vi "ma_SML Data Packing (complex input) (No State).vi"(6 "reset?":bool, 7 "ma_SML Data Packing (complex input) state":T1, 8 "error in (no error)":errorcluster, 9 "%overlap":dbl format="%.2f", 10 "size":i32, 11 "x":cdb[](array[numeric]) format="%.2f") -> (0 "error out":errorcluster, 1 "data ready?":bool, 3 "y":cdb[](array[numeric]) format="%.2f", 5 "ma_SML Data Packing (complex input) state":T1)   [LabVIEW 2020, in "NI_MAPro.lvlib"]
uses:
  NI_MAPro.lvlib
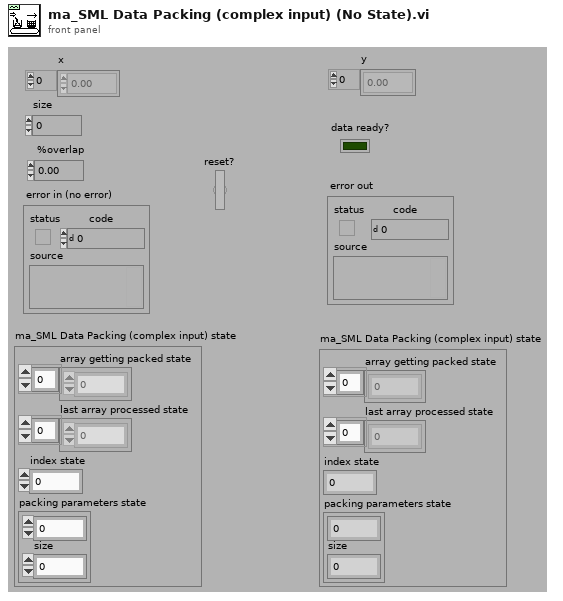
[diagram p1: front panel]
types:
  T1 = cluster{"array getting packed state":cdb[], "last array processed state":cdb[], "index state":i32, "packing parameters state":cluster{i32, "size":i32}}
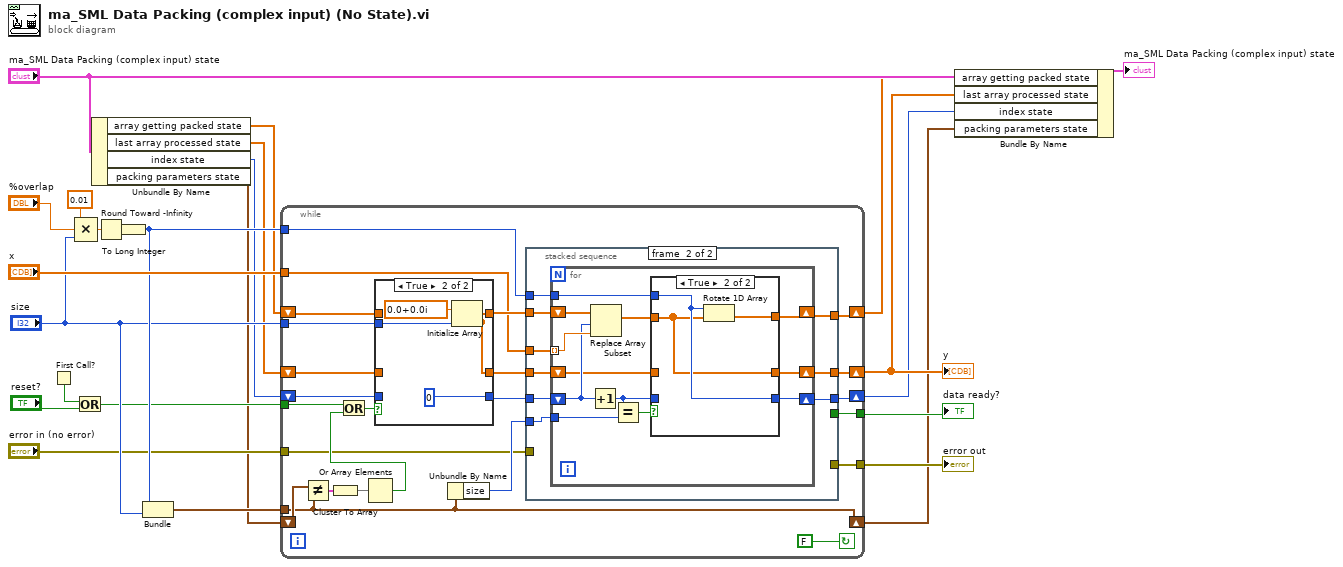
[diagram p0: block diagram]
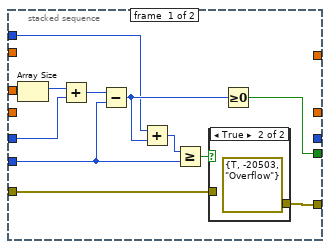
[diagram p2: hidden frame]
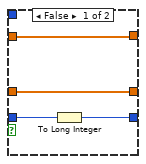
[diagram p4: hidden frame]
diagram:
  n1 = First Call?() -> (First Call?: T/F=w12:bool)
  n2 = Compound Arithmetic op=MULTIPLY(0.01, "%overlap", "size") -> (w24:dbl)
  n3 = Or(x=w12, y="reset?") -> (x .or. y?=w13:bool)
  n4 = Unbundle By Name("ma_SML Data Packing (complex input) state") -> ("array getting packed state"=w8:cdb[], "last array processed state"=w7:cdb[], "index state"=w6:i32, "packing parameters state"=w5:cluster{i32, "size":i32})
  n5 = Round Toward -Infinity(1:w24) -> (0:w21:dbl)
  n6 = To Long Integer(number=w21) -> (32bit integer=w18:i32)
  n7 = Bundle(w18, "size"="size") -> (w20:cluster{i32, "size":i32})  [unwired: 1 out]
  n8 = while {
    tunnel: "error in (no error)" -> [w25]
    tunnel: [w27] -> w14
    tunnel: w13 -> [w32]
    tunnel: [w33] -> w16
    tunnel: w18 -> [w34]
    tunnel: "x" -> [w39]
    tunnel: "size" -> [w43]
    shift-left: w6 -> [w45]
    shift-right: [w35] -> w2
    shift-left: w7 -> [w44]
    shift-right: [w37] -> w3
    shift-left: w8 -> [w42]
    shift-right: [w40] -> w4
    tunnel: w20 -> [w29]
    shift-left: w5 -> [w46]
    shift-right: [w29] -> w1
    stop <- FALSE continue-if-true
    n9 = Not Equal?(x=w46, y=w29) -> (x != y?=w48:cluster{bool, "size":bool})
    n10 = Cluster To Array(cluster=w48) -> (array=w47:bool[])
    n11 = Or Array Elements(Boolean array=w47) -> (logical OR=w31:bool)
    n12 = Or(x=w32, y=w31) -> (x .or. y?=w30:bool)
    n13 = case shown="True" w30 {
      tunnel: [w93 0] -> w36
      tunnel: w45 -> [w93 _]
      tunnel: w44 -> [w92 _]
      tunnel: [w92 w94] -> w38
      tunnel: w43 -> [_ w95]
      tunnel: [w91 w94] -> w41
      tunnel: w42 -> [w91 _]
      frame False {
      }
      frame True {
        n14 = Initialize Array(cdb 0.0+0.0i ("Element Data"), w95) -> (w94:cdb[])
      }
    }
    n15 = Unbundle By Name(w29) -> ("size"=w28:i32)
    n16 = stacked-sequence {
      tunnel: w39 -> [w60 w71]
      tunnel: w41 -> [_ w66]
      tunnel: w36 -> [w59 w67]
      tunnel: w28 -> [w53 w70]
      tunnel: [_ w68] -> w35
      tunnel: [_ w63] -> w37
      tunnel: w38 -> [_ w64]
      tunnel: [_ w65] -> w40
      tunnel: w34 -> [w50 w69]
      tunnel: [w55 _] -> w33
      tunnel: [w56 _] -> w27
      tunnel: w25 -> [w49 _]
      frame #0 {
        n17 = Array Size(array=w60) -> (size(s)=w58:i32)
        n18 = Add(x=w58, y=w59) -> (x+y=w54:i32)
        n19 = Subtract(x=w54, y=w53) -> (x-y=w51:i32)
        n20 = Add(x=w50, y=w51) -> (x+y=w52:i32)
        n21 = Greater Or Equal?(x=w52, y=w53) -> (x >= y?=w57:bool)
        n22 = case shown="True" w57 {
          tunnel: [w61 errorcluster {"status"=TRUE, "code"=-20503, "source"="Overflow"} ("error out")] -> w56
          tunnel: w49 -> [w61 _]
          frame False {
          }
          frame True {
          }
        }
        n23 = Greater Or Equal To 0?(x=w51) -> (x >= 0?=w55:bool)
      }
      frame #1 {
        n24 = for {
          tunnel: w71 -> [w83] mode=indexing
          tunnel: w70 -> [w82]
          tunnel: w69 -> [w80]
          shift-right: [w75] -> w65
          shift-left: w66 -> [w76]
          shift-right: [w78] -> w68
          shift-left: w67 -> [w77]
          shift-right: [w72] -> w63
          shift-left: w64 -> [w73]
          n25 = Increment(x=w77) -> (x+1=w81:i32)
          n26 = Replace Array Subset(array=w76, new element=w83, index=w77) -> (w79:cdb[])
          n27 = Equal?(x=w81, y=w82) -> (x = y?=w74:bool)
          n28 = case shown="True" w74 {
            tunnel: w81 -> [w87 _]
            tunnel: [w86 w89] -> w78
            tunnel: [w85 w88] -> w72
            tunnel: w73 -> [w85 _]
            tunnel: w80 -> [_ w89]
            tunnel: w79 -> [w84 w88]
            tunnel: [w84 w90] -> w75
            frame False {
              n29 = To Long Integer(number=w87) -> (32bit integer=w86:i32)
            }
            frame True {
              n30 = Rotate 1D Array(1:w88, 2:w89) -> (0:w90:cdb[])
            }
          }
        }
      }
    }
  }
  "y" <- w3
  "data ready?" <- w16
  "error out" <- w14
  n31 = Bundle By Name(cluster="ma_SML Data Packing (complex input) state", "array getting packed state"=w4, "last array processed state"=w3, "index state"=w2, "packing parameters state"=w1) -> (→"ma_SML Data Packing (complex input) state":T1)
